vi "FPGA_DMAWriteConfig.vi"(6 "SampleClock":T5, 7 "Operation":T6, 8 "error in (no error)":errorcluster, 9 "Enable":T7, 10 "Pause":bool=TRUE, 11 "DMADevRef":T8) -> (0 "error out":errorcluster, 3 "DMADevRef":T8)   [LabVIEW 2017]
uses:
  <vilib>/Rock Robotics/SystemInterfaces/DMA/FPGA_DMADevRef.ctl
  <vilib>/Rock Robotics/SystemInterfaces/DMA/FPGA_DMAEnable.ctl
  <vilib>/Rock Robotics/SystemInterfaces/DMA/FPGA_DMAWriteConfigOperation.ctl
  <vilib>/Rock Robotics/SystemInterfaces/CounterEncoderSourceConvertion/FPGA_CounterEncoderSourceConvertionLVSourceType.ctl
  <vilib>/Rock Robotics/SystemInterfaces/DIO/FPGA_DIODigitalSourceChannel.ctl
  <vilib>/Rock Robotics/SystemInterfaces/AnalogTrigger/FPGA_AnalogTriggerIndex.ctl
  <vilib>/Rock Robotics/SystemInterfaces/AnalogTrigger/FPGA_AnalogTriggerOutType.ctl
  <vilib>/Rock Robotics/SystemInterfaces/System/FPGA_SystemFPGA Ref Global.vi
  <vilib>/Utility/error.llb/Error Cluster From Error Code.vi
  <vilib>/rvi/errors/niLvFpgaAdjustHostInterfaceError.vi
  <vilib>/rvi/interface/nirviReadWriteControl/nirviReadWriteControl.xnode
  <vilib>/Rock Robotics/SystemInterfaces/System/FPGA_SystemFRC FPGA Ref.ctl
  NiFpgaLv.dll
  <vilib>/rvi/interface/Simulation/niFpgaSimulationCallBeginRW.vi
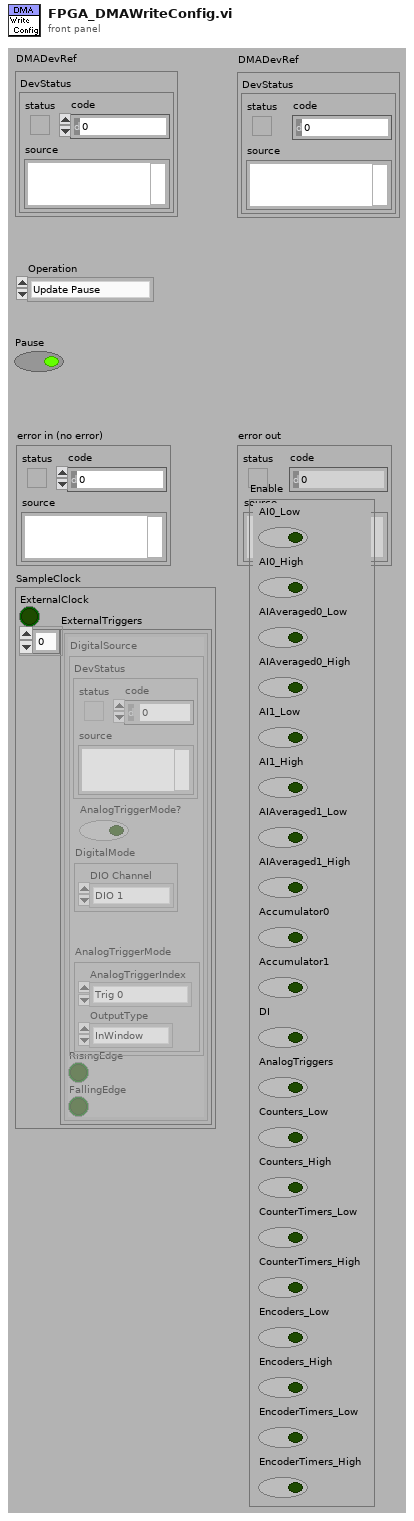
[diagram p1: front panel]
types:
  T1 = typedef "FPGA_CounterEncoderSourceConvertionLVSourceType.ctl" = cluster{"DevStatus":errorcluster, "AnalogTriggerMode?":bool, "DigitalMode":cluster{"DIO Channel":T2}, "AnalogTriggerMode":cluster{"AnalogTriggerIndex":T3, "OutputType":T4}}
  T2 = typedef "FPGA_DIODigitalSourceChannel.ctl" = enum8{"DIO 0", "DIO 1", "DIO 2", "DIO 3", "DIO 4", "DIO 5", "DIO 6", "DIO 7", "DIO 8", "DIO 9", "DIO MXP 0", "DIO MXP 1", "DIO MXP 2", "DIO MXP 3", "DIO MXP 4", "DIO MXP 5", "DIO MXP 6", "DIO MXP 7", "DIO MXP 8", "DIO MXP 9", "DIO MXP 10", "DIO MXP 11", "DIO MXP 12", "DIO MXP 13", "DIO MXP 14", "DIO MXP 15", "Disabled"}
  T3 = typedef "FPGA_AnalogTriggerIndex.ctl" = enum8{"Trig 0", "Trig 1", "Trig 2", "Trig 3", "Trig 4", "Trig 5", "Trig 6", "Trig 7", "Invalid"}
  T4 = typedef "FPGA_AnalogTriggerOutType.ctl" = enum16{"InWindow", "TriggerState", "Rising", "Falling"}
  T5 = cluster{"ExternalClock":bool, "ExternalTriggers":cluster{"DigitalSource":T1, "RisingEdge":bool, "FallingEdge":bool}[]}
  T6 = typedef "FPGA_DMAWriteConfigOperation.ctl" = enum16{"Update Pause", "Update Enable", "Update SampleClock"}
  T7 = typedef "FPGA_DMAEnable.ctl" = cluster{"AI0_Low":bool, "AI0_High":bool, "AIAveraged0_Low":bool, "AIAveraged0_High":bool, "AI1_Low":bool, "AI1_High":bool, "AIAveraged1_Low":bool, "AIAveraged1_High":bool, "Accumulator0":bool, "Accumulator1":bool, "DI":bool, "AnalogTriggers":bool, "Counters_Low":bool, "Counters_High":bool, "CounterTimers_Low":bool, "CounterTimers_High":bool, "Encoders_Low":bool, "Encoders_High":bool, "EncoderTimers_Low":bool, "EncoderTimers_High":bool}
  T8 = typedef "FPGA_DMADevRef.ctl" = cluster{"DevStatus":errorcluster}
  T9 = typedef "FPGA_SystemFRC FPGA Ref.ctl" = refnum<k20>
  T10 = cluster{"Pause":bool, "Enable":cluster{"AI0_Low":bool, "AI0_High":bool, "AIAveraged0_Low":bool, "AIAveraged0_High":bool, "AI1_Low":bool, "AI1_High":bool, "AIAveraged1_Low":bool, "AIAveraged1_High":bool, "Accumulator0":bool, "Accumulator1":bool, "DI":bool, "AnalogTriggers":bool, "Counters_Low":bool, "Counters_High":bool, "CounterTimers_Low":bool, "CounterTimers_High":bool, "Encoders_Low":bool, "Encoders_High":bool, "EncoderTimers_Low":bool, "EncoderTimers_High":bool}, "ExternalClock":bool}
  T11 = cluster{"ExternalClockSource":cluster{"Channel":fxp<+,4,4>, "Module":fxp<+,1,1>, "AnalogTrigger":bool}, "RisingEdge":bool, "FallingEdge":bool}[]
  T12 = cluster{"ExternalClockSource":cluster{"Channel":fxp<+,4,4>, "Module":fxp<+,1,1>, "AnalogTrigger":bool}, "RisingEdge":bool, "FallingEdge":bool}
  T13 = cluster{"DigitalSource":T1, "RisingEdge":bool, "FallingEdge":bool}[]
  T14 = cluster{"Channel":fxp<+,4,4>, "Module":fxp<+,1,1>, "AnalogTrigger":bool}
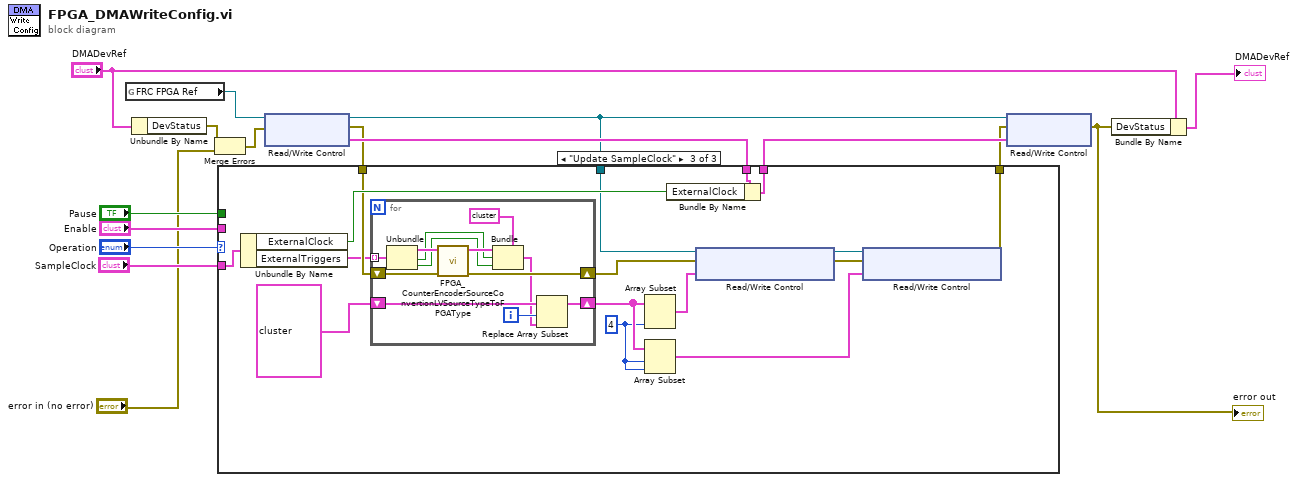
[diagram p0: block diagram]
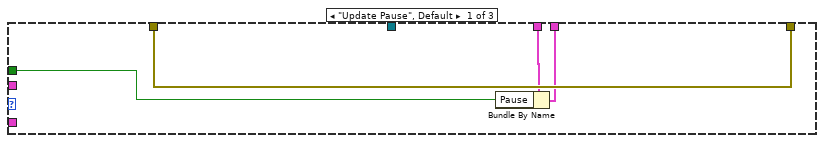
[diagram p2: hidden frame]
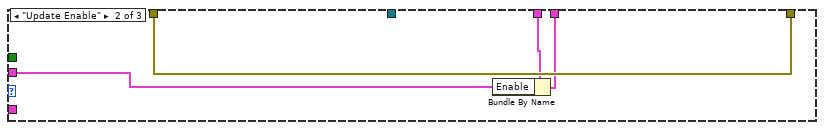
[diagram p3: hidden frame]
diagram:
  n1 = global read "FPGA_SystemFPGA Ref Global.vi" "FRC FPGA Ref"() -> (w4:T9)
  n2 = Unbundle By Name("DMADevRef") -> ("DevStatus"=w2:errorcluster)
  n3 = Merge Errors(w2, "error in (no error)") -> (w1:errorcluster)
  n4 = xnode "Read/Write Control"("FPGA VI Reference In"=w4, "error in"=w1) -> ("FPGA VI Reference Out"=w5:T9, "error out"=w7:errorcluster, "DMA.Config"=w9:T10)
  n5 = case shown="\"Update SampleClock\"" "Operation" {
    tunnel: w9 -> [w19 w23 w40]
    tunnel: [w18 w22 w39] -> w8
    tunnel: "SampleClock" -> [_ _ w38]
    tunnel: w7 -> [w20 w24 w34]
    tunnel: [w20 w24 w31] -> w6
    tunnel: "Enable" -> [_ w21 _]
    tunnel: "Pause" -> [w17 _ _]
    tunnel: w5 -> [_ _ w35]
    frame "Update Pause", Default {
      n6 = Bundle By Name(cluster=w19, "Pause"=w17) -> (w18:T10)
    }
    frame "Update Enable" {
      n7 = Bundle By Name(cluster=w23, "Enable"=w21) -> (w22:T10)
    }
    frame "Update SampleClock" {
      w26 = 4 ("length")
      n8 = Unbundle By Name(w38) -> ("ExternalClock"=w37:bool, "ExternalTriggers"=w33:T13)
      n9 = for {
        shift-right: [w52] -> w36
        shift-left: w34 -> [w51]
        tunnel: w33 -> [w50] mode=indexing
        shift-right: [w42] -> w27
        shift-left: T11 [{"ExternalClockSource"={"Channel"=0.0, "Module"=0.0, "AnalogTrigger"=FALSE}, "RisingEdge"=FALSE, "FallingEdge"=FALSE}, {"ExternalClockSource"={"Channel"=0.0, "Module"=0.0, "AnalogTrigger"=FALSE}, "RisingEdge"=FALSE, "FallingEdge"=FALSE}, {"ExternalClockSource"={"Channel"=0.0, "Module"=0.0, "AnalogTrigger"=FALSE}, "RisingEdge"=FALSE, "FallingEdge"=FALSE}, {"ExternalClockSource"={"Channel"=0.0, "Module"=0.0, "AnalogTrigger"=FALSE}, "RisingEdge"=FALSE, "FallingEdge"=FALSE}, {"ExternalClockSource"={"Channel"=0.0, "Module"=0.0, "AnalogTrigger"=FALSE}, "RisingEdge"=FALSE, "FallingEdge"=FALSE}, {"ExternalClockSource"={"Channel"=0.0, "Module"=0.0, "AnalogTrigger"=FALSE}, "RisingEdge"=FALSE, "FallingEdge"=FALSE}, {"ExternalClockSource"={"Channel"=0.0, "Module"=0.0, "AnalogTrigger"=FALSE}, "RisingEdge"=FALSE, "FallingEdge"=FALSE}, {"ExternalClockSource"={"Channel"=0.0, "Module"=0.0, "AnalogTrigger"=FALSE}, "RisingEdge"=FALSE, "FallingEdge"=FALSE}] ("DMA.ExternalTriggers") -> [w43]
        i -> [w44]
        n10 = Unbundle(w50) -> ("DigitalSource"=w49:T1, "RisingEdge"=w47:bool, "FallingEdge"=w46:bool)
        n11 = call <vilib>:"FPGA_CounterEncoderSourceConvertionLVSourceTypeToFPGAType.vi"("error in (no error)"=w51, "DigitalSource"=w49) -> ("error out"=w52:errorcluster, "FPGASource"=w48:T14)  [unwired: 8 out]
        n12 = Bundle(cluster=T12 {"ExternalClockSource"={"Channel"=0.0, "Module"=0.0, "AnalogTrigger"=FALSE}, "RisingEdge"=TRUE, "FallingEdge"=FALSE} ("Trigger"), "ExternalClockSource"=w48, "RisingEdge"=w47, "FallingEdge"=w46) -> (w41:T12)
        n13 = Replace Array Subset(array=w43, new element=w41, index=w44) -> (w42:T11)
      }
      n14 = Array Subset(array=w27, length=w26) -> (w28:T11)  [unwired: 1 in]
      n15 = Array Subset(array=w27, index=w26, length=w26) -> (w25:T11)
      n16 = Bundle By Name(cluster=w40, "ExternalClock"=w37) -> (w39:T10)
      n17 = xnode "Read/Write Control"("FPGA VI Reference In"=w35, "error in"=w36, "DMA.ExternalTriggers0"=w28) -> ("FPGA VI Reference Out"=w29:T9, "error out"=w30:errorcluster)
      n18 = xnode "Read/Write Control"("FPGA VI Reference In"=w29, "error in"=w30, "DMA.ExternalTriggers1"=w25) -> ("error out"=w31:errorcluster)  [unwired: 1 out]
    }
  }
  n19 = xnode "Read/Write Control"("FPGA VI Reference In"=w5, "error in"=w6, "DMA.Config"=w8) -> ("error out"=w14:errorcluster)  [unwired: 1 out]
  "error out" <- w14
  n20 = Bundle By Name(cluster="DMADevRef", "DevStatus"=w14) -> (→"DMADevRef":T8)
